vi "Format Word for CSV.vi"(8 "error in":errorcluster, 10 "data word format":T1="Hexadecimal", 11 "Word":T2 {"type" format="%04x"; "activity" format="%04x"; "error" format="%04x"; "cwd1" format="%04x"; "cwd2" format="%04x"; "swd1" format="%04x"; "swd2" format="%04x"; "data" format="%04x"}) -> (0 "error out":errorcluster, 3 "String Array":string[](array[string]))   [LabVIEW 2020, in "Ballard MIL-STD-1553 Engine.lvlib" / "Implementation.lvlib" / "CSV Word Logger.lvclass"]
uses:
  CSV Word Logger.lvclass
  Word.ctl
  Shared/Data Word Format.ctl
  Rx Execution Unit/Rx Execution Unit.lvclass
  <instrlib>/BTI1553Lib/BTI1553LV.lvlib
  Implementation.lvlib
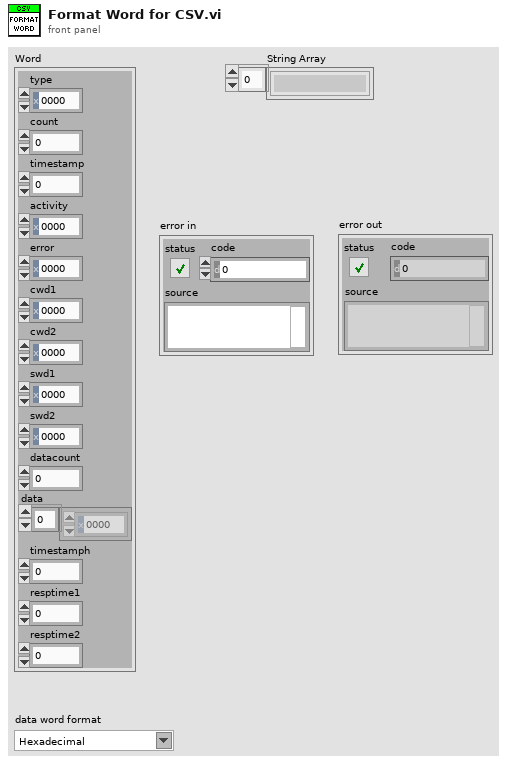
[diagram p1: front panel]
types:
  T1 = typedef "Data Word Format.ctl" = string
  T2 = typedef "Ballard MIL-STD-1553 Engine.lvlib/Implementation.lvlib/Word.ctl" = cluster{"type":u16, "count":u16, "timestamp":u32, "activity":u16, "error":u16, "cwd1":u16, "cwd2":u16, "swd1":u16, "swd2":u16, "datacount":u16, "data":u16[], "timestamph":u32, "resptime1":u16, "resptime2":u16}
  T3 = typedef "BTI1553LV.lvlib/1553 Activity Flags.ctl" = cluster{"channelnumber":i32, "transmittedcwd1":bool, "transmittedcwd2":bool, "transmittedswd1":bool, "transmittedswd2":bool, "receivedcwd1":bool, "receivedcwd2":bool, "receivedswd1":bool, "receivedswd2":bool, "transmitteddwd":bool, "receiveddwd":bool, "reserved1":i8, "reserved2":i8, "bus":u32}
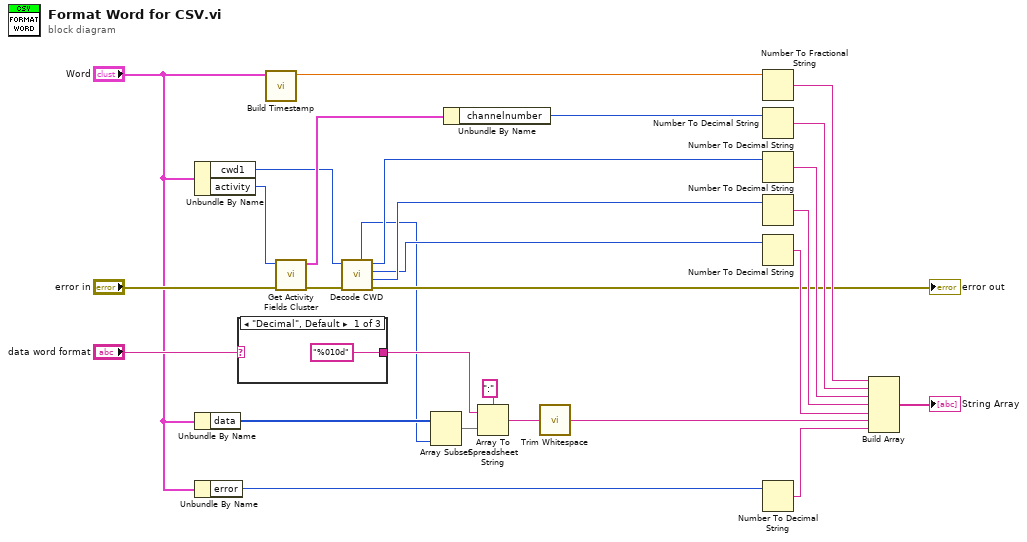
[diagram p0: block diagram]
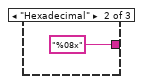
[diagram p2: hidden frame]
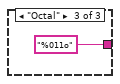
[diagram p3: hidden frame]
diagram:
  n1 = Unbundle By Name("Word") -> ("cwd1"=w16:u16, "activity"=w21:u16)
  n2 = Unbundle By Name("Word") -> ("data"=w8:u16[])
  n3 = Unbundle By Name("Word") -> ("error"=w6:u16)
  n4 = case shown="\"Decimal\", Default" "data word format" {
    tunnel: ["%010d" ("format string") "%08x" ("format string") "%011o" ("format string")] -> w11
    frame "Decimal", Default {
    }
    frame "Hexadecimal" {
    }
    frame "Octal" {
    }
  }
  n5 = call "Build Timestamp.vi"("record"="Word") -> ("timestamp"=w22:dbl)  [unwired: 10 in]
  n6 = call <instrlib>:"Get Activity Fields Cluster.vi"("error in (no error)"="error in", "activity"=w21) -> ("error out"=w17:errorcluster, "activity flags"=w20:T3)  [unwired: 8 in]
  n7 = call <instrlib>:"Decode CWD.vi"("error in (no error)"=w17, "command word"=w16) -> ("error out"=→"error out":errorcluster, "subaddress out"=w14:i32, "transmit/receive bit value out"=w13:i32, "terminal address out"=w15:i32, "word count out"=w5:i32)  [unwired: 5 in]
  n8 = Array Subset(array=w8, length=w5) -> (w7:u16[])  [unwired: 1 in]
  n9 = Unbundle By Name(w20) -> ("channelnumber"=w19:i32)
  n10 = Array To Spreadsheet String(delimiter (Tab)=":", array=w7, 3:w11) -> (spreadsheet string=w2:string)
  n11 = call <vilib>:"Trim Whitespace.vi"("string"=w2) -> ("trimmed string"=w1:string)  [unwired: 1 in]
  n12 = Number To Fractional String(number=w22) -> (F-format string=w27:string)  [unwired: 3 in]
  n13 = Number To Decimal String(number=w19) -> (decimal integer string=w24:string)  [unwired: 1 in]
  n14 = Number To Decimal String(number=w15) -> (decimal integer string=w26:string)  [unwired: 1 in]
  n15 = Number To Decimal String(number=w14) -> (decimal integer string=w25:string)  [unwired: 1 in]
  n16 = Number To Decimal String(number=w13) -> (decimal integer string=w10:string)  [unwired: 1 in]
  n17 = Number To Decimal String(number=w6) -> (decimal integer string=w3:string)  [unwired: 1 in]
  n18 = Build Array(w27, w24, w26, w25, w10, w1, w3) -> (→"String Array":string[])
